vi "loadConfig.vi"(2 "error in (no error)":errorcluster, 3 "file path (use dialog)":path) -> (0 "error out":errorcluster, 1 "text":string)   [LabVIEW 2012]
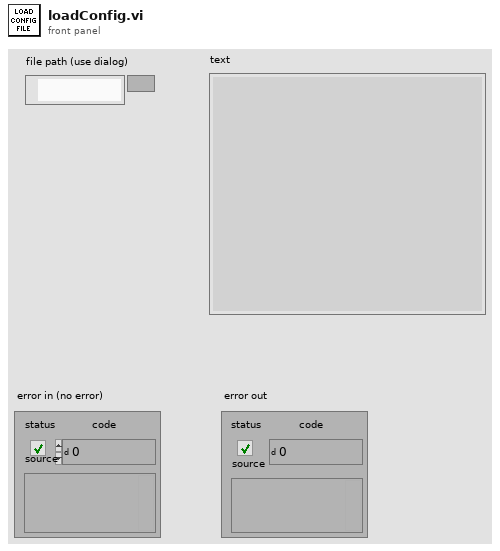
[diagram p1: front panel]
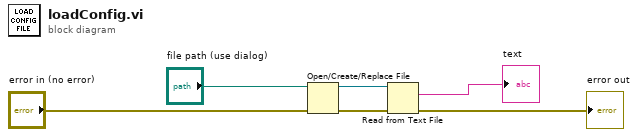
[diagram p0: block diagram]
diagram:
  n1 = Open/Create/Replace File(file path (use dialog)="file path (use dialog)", error in="error in (no error)") -> (refnum out=w6:refnum<file>, error out=w5:errorcluster)  [unwired: 4 in, 1 out]
  n2 = Read from Text File(file (use dialog)=w6, error in=w5) -> (text=→"text":string, error out=→"error out":errorcluster)  [unwired: 2 in, 2 out]
